vi "CloseFile.vi"(8 "error in (no error)":errorcluster, 11 "DataLog in":refnum<class "DataLog.lvclass">) -> (0 "error out":errorcluster, 3 "DataLog out":refnum<class "DataLog.lvclass">)   [LabVIEW 2018, in "DataLog.lvclass"]
uses:
  DataLog.lvclass
  DataLog.lvclass/DataLog.ctl
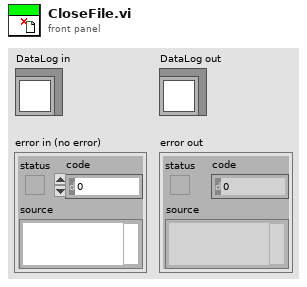
[diagram p1: front panel]
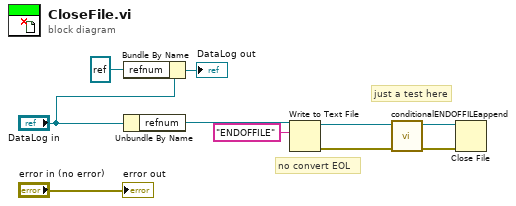
[diagram p0: block diagram]
diagram:
  # "just a test here"
  # "no convert EOL"
  n1 = Bundle By Name(cluster="DataLog in", "refnum"=refnum<file> refnum) -> (→"DataLog out":refnum<class "DataLog.lvclass">)
  n2 = Unbundle By Name("DataLog in") -> ("refnum"=w6:refnum<file>)
  n3 = Write to Text File(file (use dialog)=w6, text="ENDOFFILE") -> (refnum out=w4:refnum<file>, error out=w2:errorcluster)  [unwired: 2 in, 1 out]
  n4 = call "conditionalENDOFFILEappend.vi"("error in"=w2, "refnum"=w4) -> ("error out"=w1:errorcluster, "refnum out"=w3:refnum<file>)  [unwired: 8 in]
  n5 = Close File(refnum=w3, error in=w1) -> ()  [unwired: 2 out]
  "error out" <- "error in (no error)"
